vi "Get Magnet Vector.vi"(8 "error in (no error)":errorcluster, 11 "Instrument.VRM in":refnum<class "Instrument.OxfordVRM.lvclass">) -> (0 "error out":errorcluster, 1 "status":string, 2 "Magnet Field (T)":dbl[](array[numeric]), 3 "Instrument.VRM out":refnum<class "Instrument.OxfordVRM.lvclass">, 4 "finished":bool)   [LabVIEW 2019, in "Instrument.OxfordVRM.lvclass"]
uses:
  Instrument.OxfordVRM.lvclass
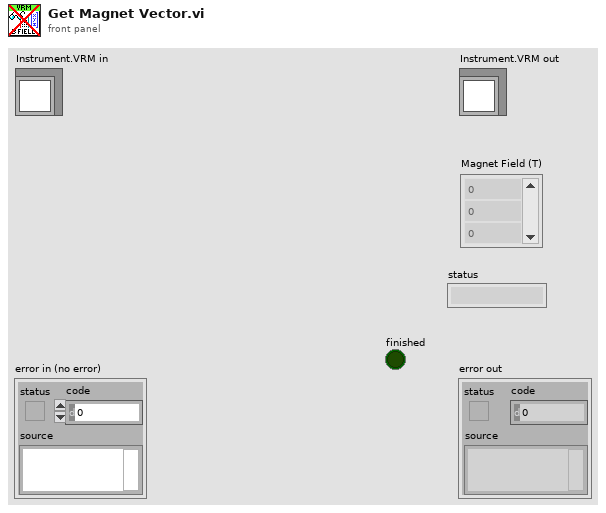
[diagram p1: front panel]
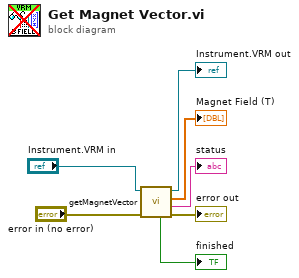
[diagram p0: block diagram]
diagram:
  n1 = call-dynamic "getMagnetVector.vi"("error in (no error)"="error in (no error)", "Instrument.VRM in"="Instrument.VRM in") -> ("error out"=→"error out":errorcluster, "status"=→"status":string, "Magnet Field (T)"=→"Magnet Field (T)":dbl[], "Instrument.VRM out"=→"Instrument.VRM out":refnum<class "Instrument.OxfordVRM.lvclass">, "finished"=→"finished":bool)  [unwired: 5 in]
